vi "CRYSet Cursor Infor.vi"(0 "This VI":refnum<vi>, 1 "Active Cursor":u32, 2 "Graph Type":string="LineStyle", 3 "XY Graph Ref":refnum<vi>, 4 "Wave Graph Ref":refnum<vi>, 5 "Intensity Graph Ref":refnum<vi>, 8 "Property Set?":bool) -> (16 "Cursor Name":string, 18 "Cursor Color":u32, 20 "CursorLineStyle":string, 21 "CursorLineWidth":string, 22 "CursorPointStyle":string, 23 "CursorStyle":string)   [LabVIEW 2013]
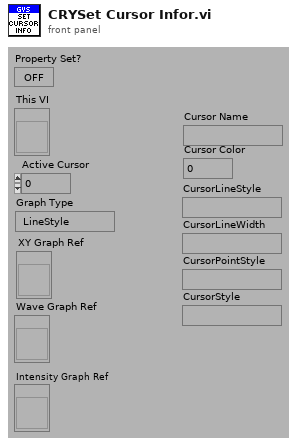
[diagram p1: front panel]
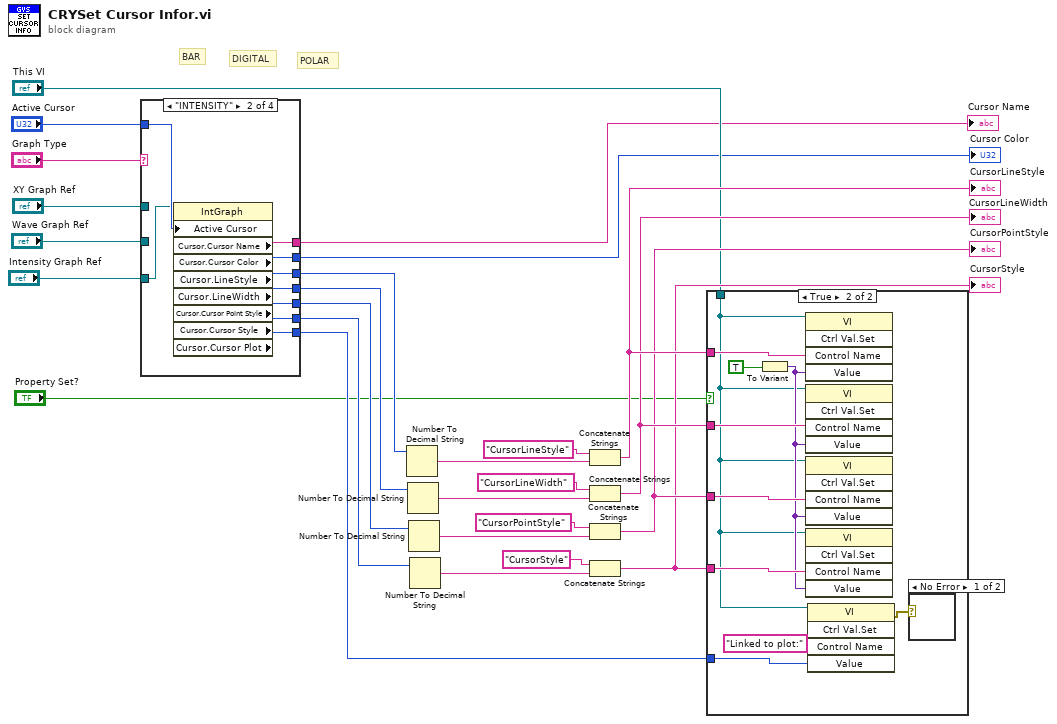
[diagram p0: block diagram]
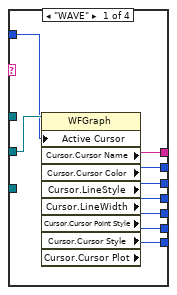
[diagram p4: hidden frame]
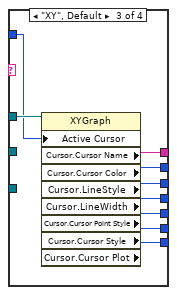
[diagram p5: hidden frame]
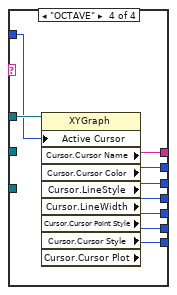
[diagram p6: hidden frame]
diagram:
  # "POLAR"
  # "DIGITAL"
  # "BAR"
  n1 = case shown="\"INTENSITY\"" "Graph Type" {
    tunnel: "XY Graph Ref" -> [_ _ w46 w55]
    tunnel: [w35 w44 w53 w62] -> w12
    tunnel: [w34 w43 w52 w61] -> w11
    tunnel: [w33 w42 w51 w60] -> w10
    tunnel: [w32 w41 w50 w59] -> w9
    tunnel: "Wave Graph Ref" -> [w28 _ _ _]
    tunnel: [w31 w40 w49 w58] -> w6
    tunnel: [w30 w39 w48 w57] -> w5
    tunnel: [w29 w38 w47 w56] -> w4
    tunnel: "Active Cursor" -> [w27 w37 w45 w54]
    tunnel: "Intensity Graph Ref" -> [_ w36 _ _]
    frame "WAVE" {
      n2 = property class="WFGraph"(reference=w28, "Active Cursor"=w27) -> ("Cursor.Cursor Name"=w31:string, "Cursor.Cursor Color"=w30:u32, "Cursor.LineStyle"=w35:u8, "Cursor.LineWidth"=w34:u8, "Cursor.Cursor Point Style"=w33:u8, "Cursor.Cursor Style"=w32:u8, "Cursor.Cursor Plot"=w29:i32)  [unwired: 1 in, 2 out]
    }
    frame "INTENSITY" {
      n3 = property class="IntGraph"(reference=w36, "Active Cursor"=w37) -> ("Cursor.Cursor Name"=w40:string, "Cursor.Cursor Color"=w39:u32, "Cursor.LineStyle"=w44:u8, "Cursor.LineWidth"=w43:u8, "Cursor.Cursor Point Style"=w42:u8, "Cursor.Cursor Style"=w41:u8, "Cursor.Cursor Plot"=w38:i32)  [unwired: 1 in, 2 out]
    }
    frame "XY", Default {
      n4 = property class="XYGraph"(reference=w46, "Active Cursor"=w45) -> ("Cursor.Cursor Name"=w49:string, "Cursor.Cursor Color"=w48:u32, "Cursor.LineStyle"=w53:u8, "Cursor.LineWidth"=w52:u8, "Cursor.Cursor Point Style"=w51:u8, "Cursor.Cursor Style"=w50:u8, "Cursor.Cursor Plot"=w47:i32)  [unwired: 1 in, 2 out]
    }
    frame "OCTAVE" {
      n5 = property class="XYGraph"(reference=w55, "Active Cursor"=w54) -> ("Cursor.Cursor Name"=w58:string, "Cursor.Cursor Color"=w57:u32, "Cursor.LineStyle"=w62:u8, "Cursor.LineWidth"=w61:u8, "Cursor.Cursor Point Style"=w60:u8, "Cursor.Cursor Style"=w59:u8, "Cursor.Cursor Plot"=w56:i32)  [unwired: 1 in, 2 out]
    }
  }
  "Cursor Name" <- w6
  "Cursor Color" <- w5
  n6 = Number To Decimal String(number=w12) -> (decimal integer string=w26:string)  [unwired: 1 out]
  n7 = Number To Decimal String(number=w11) -> (decimal integer string=w25:string)  [unwired: 1 out]
  n8 = Number To Decimal String(number=w10) -> (decimal integer string=w24:string)  [unwired: 1 out]
  n9 = Number To Decimal String(number=w9) -> (decimal integer string=w23:string)  [unwired: 1 out]
  n10 = Concatenate Strings("CursorLineStyle", w26) -> (w18:string)
  "CursorLineStyle" <- w18
  n11 = Concatenate Strings("CursorLineWidth", w25) -> (w17:string)
  "CursorLineWidth" <- w17
  n12 = Concatenate Strings("CursorPointStyle", w24) -> (w16:string)
  "CursorPointStyle" <- w16
  n13 = Concatenate Strings("CursorStyle", w23) -> (w15:string)
  "CursorStyle" <- w15
  n14 = case shown="True" "Property Set?" {
    tunnel: w18 -> [_ w72]
    tunnel: w17 -> [_ w71]
    tunnel: w16 -> [_ w70]
    tunnel: w15 -> [_ w69]
    tunnel: "This VI" -> [_ w66]
    tunnel: w4 -> [_ w64]
    frame False {
    }
    frame True {
      n15 = To Variant(anything=TRUE) -> (Variant=w67:variant)
      n16 = invoke class="VI" method="Ctrl Val.Set"(reference=w66, "Control Name"=w72, "Value"=w67) -> ()  [unwired: 2 in, 5 out]
      n17 = invoke class="VI" method="Ctrl Val.Set"(reference=w66, "Control Name"=w71, "Value"=w67) -> ()  [unwired: 2 in, 5 out]
      n18 = invoke class="VI" method="Ctrl Val.Set"(reference=w66, "Control Name"=w70, "Value"=w67) -> ()  [unwired: 2 in, 5 out]
      n19 = invoke class="VI" method="Ctrl Val.Set"(reference=w66, "Control Name"=w69, "Value"=w67) -> ()  [unwired: 2 in, 5 out]
      n20 = invoke class="VI" method="Ctrl Val.Set"(reference=w66, "Control Name"="Linked to plot:", "Value"=w64) -> (error out=w63:errorcluster)  [unwired: 2 in, 4 out]
      n21 = case shown="No Error" w63 {
        frame No Error {
        }
        frame Error {
        }
      }
    }
  }
